vi "Write Scale.vi"(10 "ConfigScale":T1={"scale [EU/RAW]"=1.0, "offset [EU]"=0.0} {"offset [EU]" format="%0.2f"; "scale [EU/RAW]" format="%0.2f"}, 11 "Sig_AI in":refnum<class "Sig_AI.lvclass">) -> (3 "Sig_AI out":refnum<class "Sig_AI.lvclass">)   [LabVIEW 2019, in "Sig_AI.lvclass"]
uses:
  Sig_AI.lvclass
  TypeDef/Config_Scale.ctl
  Sig_AI.lvclass/Sig_AI.ctl
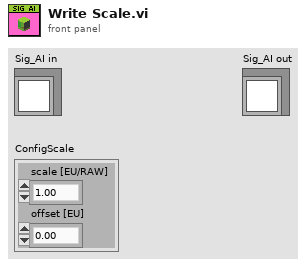
[diagram p1: front panel]
types:
  T1 = typedef "Config_Scale.ctl" = cluster{"scale [EU/RAW]":dbl, "offset [EU]":dbl}
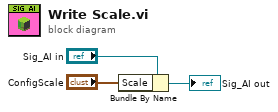
[diagram p0: block diagram]
diagram:
  n1 = Bundle By Name(cluster="Sig_AI in", "Scale"="ConfigScale") -> (→"Sig_AI out":refnum<class "Sig_AI.lvclass">)
